vi "AG State Controller.vi"(7 "queue Ref":refnum<queue>, 9 "Error In":errorcluster, 10 "Default State":T1) -> (1 "Error Out":errorcluster, 2 "State Out":T1, 4 "New State":bool)   [LabVIEW 2012]
doc: "Control a state machine based on the myDAQ State control\n\nBehavior\n1. Check the queue for new elements (Timeout = 0)\n2. If timeout use the default state\n3. If there is an error override other states and go to the error state."
uses:
  <userlib>/H_Utilities/myDAQ_State.ctl
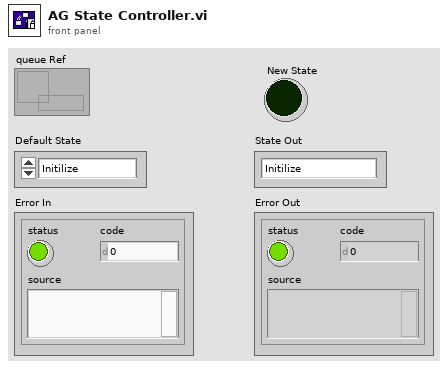
[diagram p1: front panel]
types:
  T1 = typedef "myDAQ_State.ctl" = enum16{"Initilize", "Connect", "Calibrate", "Communicate", "Wait", "Disconnect", "Error", "Close"}
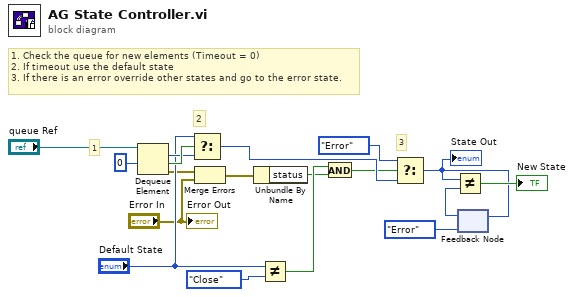
[diagram p0: block diagram]
diagram:
  # "3"
  # "2"
  # "1"
  # "1. Check the queue for new elements (Timeout = 0)\n2. If timeout use the default state\n3. If there is an error override other states and go to the error state."
  n1 = Dequeue Element(queue="queue Ref", timeout in ms (-1)=0) -> (element=w17:T1, timed out?=w18:bool, error out=w2:errorcluster)  [unwired: 1 in, 1 out]
  n2 = Select(t="Default State", s=w18, f=w17) -> (s? t:f=w9:T1)
  n3 = Merge Errors(w2, "Error In") -> (w1:errorcluster)
  n4 = Unbundle By Name(w1) -> ("status"=w6:bool)
  n5 = Not Equal?(x="Default State", y=myDAQ_State."Close") -> (x != y?=w7:bool)
  n6 = And(x=w7, y=w6) -> (x .and. y?=w5:bool)
  n7 = Select(t=myDAQ_State."Error", s=w5, f=w9) -> (s? t:f=w10:T1)
  "State Out" <- w10
  n8 = feedback-in #1(w10) -> ()
  n9 = feedback #1(myDAQ_State."Error" ("t")) -> (w12:T1)
  n10 = Not Equal?(x=w10, y=w12) -> (x != y?=→"New State":bool)
  "Error Out" <- "Error In"
